vi "Show Report.vi"(8 "error in (no error)":errorcluster, 11 "IMAQ Display in":refnum<class "HIJ Vision Display.lvclass">) -> (0 "error out":errorcluster, 3 "IMAQ Display out":refnum<class "HIJ Vision Display.lvclass">)   [LabVIEW 2014, in "HIJ Vision Display.lvlib" / "HIJ Vision Display.lvclass"]
uses:
  HIJ Vision Display.lvclass
  HIJ Vision Display.lvclass/HIJ Vision Display.ctl
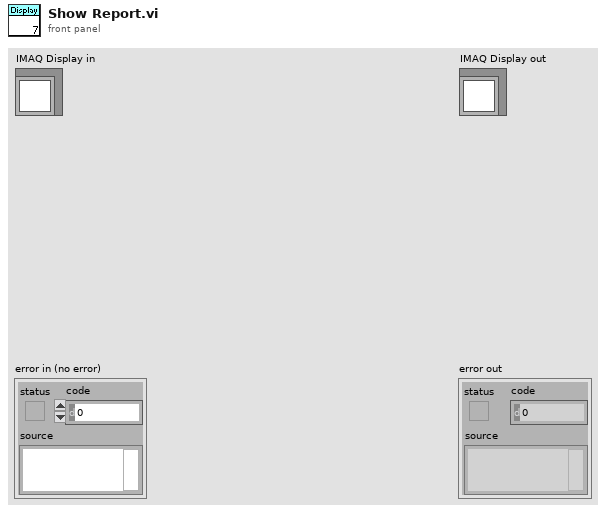
[diagram p1: front panel]
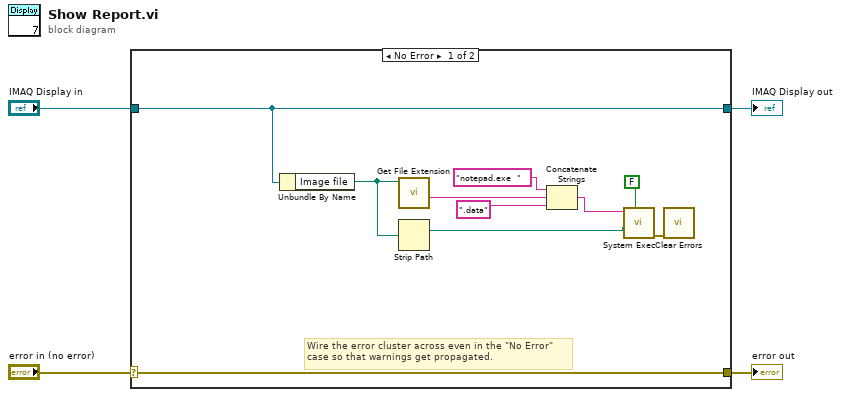
[diagram p0: block diagram]
diagram:
  n1 = case shown="No Error" "error in (no error)" {
    selector: "error in (no error)" -> [w14 w16]
    tunnel: [w14 w16] -> w3
    tunnel: [w5 w15] -> w1
    tunnel: "IMAQ Display in" -> [w5 w15]
    frame No Error {
      # "Wire the error cluster across even in the \"No Error\"\ncase so that warnings get propagated."
      n2 = Unbundle By Name(w5) -> ("Image file"=w6:path)
      n3 = call <vilib>:"Get File Extension.vi"("file"=w6) -> ("filename without extension"=w10:string)  [unwired: 7 in, 3 out]
      n4 = Strip Path(path=w6) -> (stripped path=w11:path)  [unwired: 1 out]
      n5 = Concatenate Strings("notepad.exe  " ("command line"), w10, ".data" ("string")) -> (w12:string)
      n6 = call <vilib>:"System Exec.vi"("wait until completion? (T)"=FALSE, "working directory"=w11, "command line"=w12) -> ("error out"=w9:errorcluster)  [unwired: 5 in, 3 out]
      n7 = call <vilib>:"Clear Errors.vi"("error in (no error)"=w9) -> ()  [unwired: 5 in, 2 out]
    }
    frame Error {
    }
  }
  "error out" <- w3
  "IMAQ Display out" <- w1
